vi "Lookup Chart Manager.vi"(8 "error in (no error)":errorcluster, 11 "HistorianCharting in":refnum<class "HistorianCharting.lvclass">) -> (0 "error out":errorcluster, 3 "HistorianCharting out":refnum<class "HistorianCharting.lvclass">)   [LabVIEW 2020, in "VolatusGUIElements.lvlib" / "HistorianCharting.lvclass"]
uses:
  HistorianCharting.lvclass
  HistorianCharting.lvclass/HistorianCharting.ctl
  Volatus/VolatusAPI/VolatusAPI.lvclass
  VolatusGUI/Historian Charting Manager ID/Historian Charting Manager ID.lvclass
  C:/dev/lv20CE/relink/lv-volatus/VolatusGUI/Historian Charting Manager ID/Historian Charting Manager ID.lvclass
  C:/dev/lv20CE/relink/lv-volatus/Volatus/Identity/Identity.lvclass
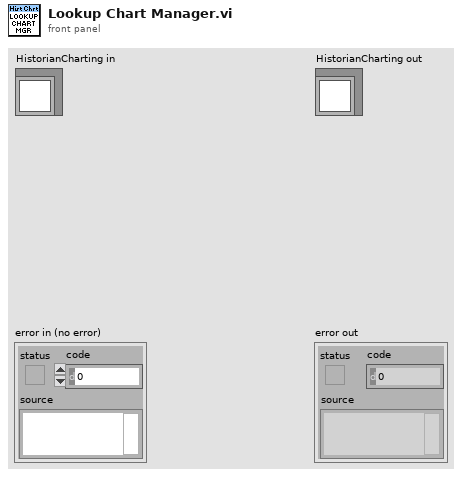
[diagram p1: front panel]
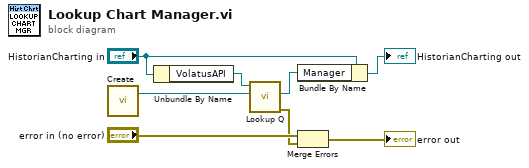
[diagram p0: block diagram]
diagram:
  n1 = call "Create.vi"() -> ("Historian Charting Manager ID out"=w7:refnum<class "Historian Charting Manager ID.lvclass">)  [unwired: 7 in]
  n2 = Unbundle By Name("HistorianCharting in") -> ("VolatusAPI"=w5:refnum<class "VolatusAPI.lvclass">)
  n3 = call "Lookup Q.vi"("Identity"=w7, "VolatusAPI in"=w5) -> ("error out"=w1:errorcluster, "MessageQ"=w3:refnum<class "MessageQ.lvclass">)  [unwired: 7 in, 1 out]
  n4 = Bundle By Name(cluster="HistorianCharting in", "Manager"=w3) -> (→"HistorianCharting out":refnum<class "HistorianCharting.lvclass">)
  n5 = Merge Errors("error in (no error)", w1) -> (→"error out":errorcluster)
